vi "cul gantry position.vi"(10 "position in":dbl[](array[numeric])=[3.0, 3.0, 3.0, 3.0], 11 "Origin and Axis path":path=path "D:/Gantry_General/Main/ms_kao/gantry path/path data/Origin and Axis position.txt") -> (2 "position out":dbl[](array[numeric]))   [LabVIEW 2016]
uses:
  <vilib>/Utility/file.llb/Read Delimited Spreadsheet (DBL).vi
panel:
  out "angle degress":dbl
  out "all rows":dbl[][](array[numeric])
  out "Origin":dbl[](array[numeric])
  out "angle radian":dbl
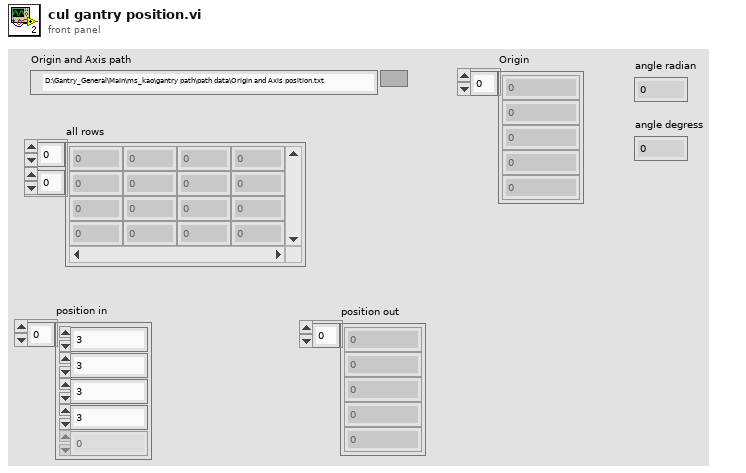
[diagram p1: front panel]
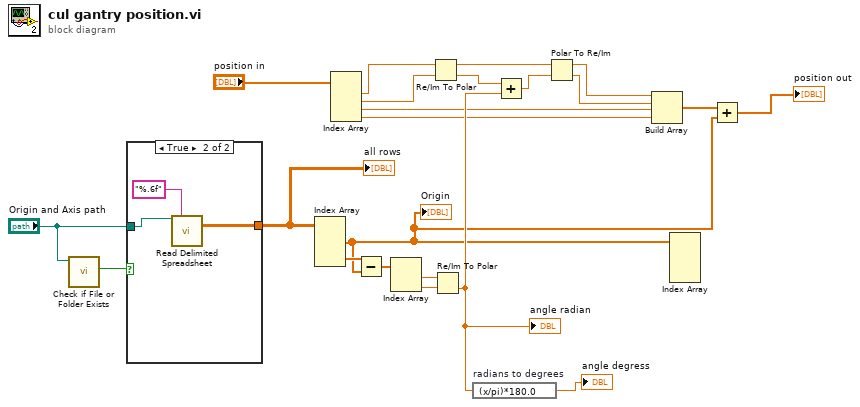
[diagram p0: block diagram]
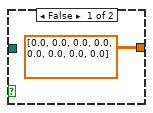
[diagram p2: hidden frame]
diagram:
  n1 = call <vilib>:"Check if File or Folder Exists.vi"("path"="Origin and Axis path") -> ("file or folder exists?"=w15:bool)  [unwired: 8 in, 2 out]
  n2 = case shown="True" w15 {
    tunnel: [dbl[][] [[0.0, 0.0, 0.0, 0.0], [0.0, 0.0, 0.0, 0.0]] ("all rows") w26] -> w18
    tunnel: "Origin and Axis path" -> [_ w25]
    frame False {
    }
    frame True {
      n3 = call-poly <vilib>:"Read Delimited Spreadsheet.vi"("file path (dialog if empty)"=w25, "format (%.3f)"="%.6f") -> ("all rows"=w26:dbl[][])  [unwired: 8 in, 5 out]
    }
  }
  "all rows" <- w18
  n4 = Index Array(array=w18) -> (element #1=w3:dbl[], element #2=w20:dbl[])  [unwired: 4 in]
  "Origin" <- w3
  n5 = Index Array(array="position in") -> (element #1=w6:dbl, element #2=w5:dbl, element #3=w1:dbl, element #4=w2:dbl)  [unwired: 4 in]
  n6 = Subtract(x=w20, y=w3) -> (x-y=w19:dbl[])
  n7 = Index Array(array=w19) -> (element #1=w22:dbl, element #2=w21:dbl)  [unwired: 2 in]
  n8 = Re/Im To Polar(2:w5, 3:w6) -> (0:w13:dbl, 1:w11:dbl)
  n9 = Re/Im To Polar(2:w21, 3:w22) -> (0:w14:dbl)  [unwired: 1 out]
  "angle radian" <- w14
  n10 = expression code="(x/pi)*180.0" "radians to degrees"(w14) -> (→"angle degress":dbl)
  n11 = Add(x=w13, y=w14) -> (x+y=w12:dbl)
  n12 = Polar To Re/Im(2:w12, 3:w11) -> (0:w9:dbl, 1:w10:dbl)
  n13 = Build Array(w10, w9, w1, w2) -> (w4:dbl[])
  n14 = Index Array(array=w3) -> ()  [unwired: 4 in, 4 out]
  n15 = Add(x=w4, y=w3) -> (x+y=→"position out":dbl[])
